vi "Timer.vi"() -> ()   [LabVIEW 2023]
panel:
  out "Output":dbl format="%.1f"
  in  "Length":dbl
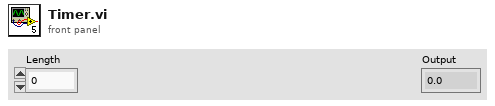
[diagram p1: front panel]
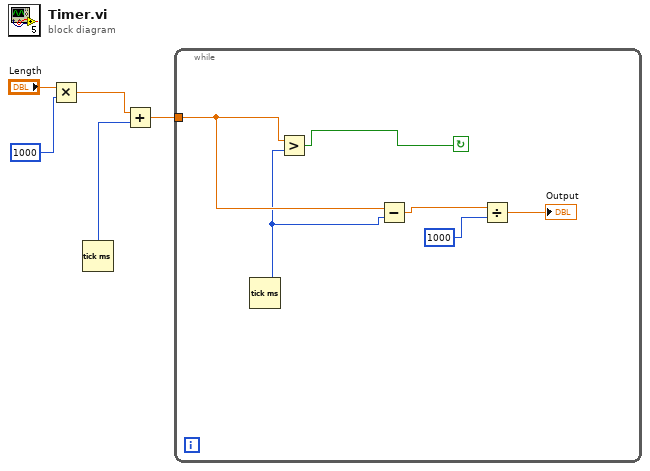
[diagram p0: block diagram]
diagram:
  n1 = Multiply(x="Length", y=1000) -> (x*y=w3:dbl)
  n2 = Tick Count (ms)() -> (millisecond timer value=w2:u32)
  n3 = Add(x=w3, y=w2) -> (x+y=w1:dbl)
  n4 = while {
    tunnel: w1 -> [w10]
    stop <- w11 continue-if-true
    n5 = Tick Count (ms)() -> (millisecond timer value=w9:u32)
    n6 = Greater?(x=w10, y=w9) -> (0:w11:bool)
    n7 = Subtract(x=w10, y=w9) -> (x-y=w8:dbl)
    n8 = Divide(x=w8, y=1000) -> (x/y=→"Output":dbl)
  }
